vi "MoveMirror.vi"(1 "error in 2":errorcluster, 3 "POS X rad":dbl, 4 "POS Y rad":dbl) -> (0 "error out 2":errorcluster)   [LabVIEW 2011]
uses:
  Utilities/controls/ctlSeqFNs_PI_SysNr.ctl
  Variables/GlobalSetConfigurationPhysikalInstruments.vi
  Variables/GlobalSetNumberOfDigits_PhysikalInstruments.vi
  Variables/GlobalSetGetPositionParameters.vi
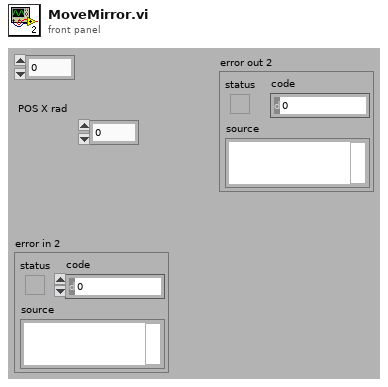
[diagram p1: front panel]
types:
  T1 = typedef "ctlSeqFNs_PI_SysNr.ctl" = enum16{"Zero", "E517", "E710"}
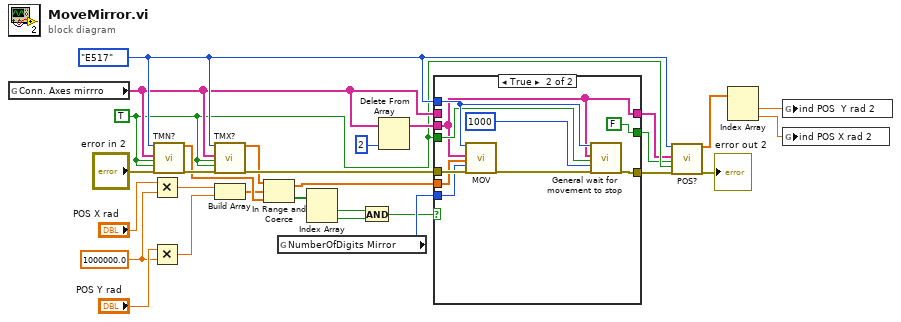
[diagram p0: block diagram]
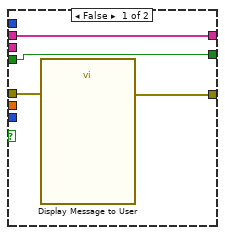
[diagram p2: hidden frame]
diagram:
  w15 = 1000000.0 ("y")
  w3 = TRUE ("All axes?")
  w9 = ctlSeqFNs_PI_SysNr."E517" ("DeviceNr.")
  n1 = global read "GlobalSetConfigurationPhysikalInstruments.vi" "Conn. Axes mirrro"() -> (w5:string[])
  n2 = Multiply(x="POS X rad", y=w15) -> (x*y=w13:dbl)
  n3 = Multiply(x="POS Y rad", y=w15) -> (x*y=w16:dbl)
  n4 = call "TMN?.vi"("System no."=w9, "Axes to query"=w5, "All axes?"=w3, "Axis identifier?"=w3, "error in"="error in 2") -> ("Minimum travel limit"=w25:dbl[], "error out"=w28:errorcluster)  [unwired: 13 in]
  n5 = call "TMX?.vi"("System no."=w9, "Axes to query"=w5, "All axes?"=w3, "Axis identifier?"=w3, "error in"=w28) -> ("Maximum travel limit"=w24:dbl[], "error out"=w27:errorcluster)  [unwired: 13 in]
  n6 = Build Array(w13, w16) -> (w23:dbl[])
  n7 = In Range and Coerce(upper limit=w24, x=w23, lower limit=w25) -> (coerced(x)=w18:dbl[], In Range?=w22:bool[])
  n8 = global read "GlobalSetNumberOfDigits_PhysikalInstruments.vi" "NumberOfDigits Mirror"() -> (w26:i32)
  n9 = Index Array(array=w22) -> (element #1=w21:bool, element #2=w20:bool)  [unwired: 2 in]
  n10 = And(x=w21, y=w20) -> (x .and. y?=w19:bool)
  n11 = Delete From Array(array=w5, index=2) -> (array with subset deleted=w6:string[])  [unwired: 1 in, 1 out]
  n12 = case shown="True" w19 {
    tunnel: w18 -> [_ w37]
    tunnel: w27 -> [w32 w43]
    tunnel: [w33 w41] -> w8
    tunnel: w6 -> [_ w35]
    tunnel: w9 -> [_ w40]
    tunnel: w26 -> [_ w38]
    tunnel: w5 -> [w31 _]
    tunnel: w3 -> [w30 w36]
    tunnel: [w31 w35] -> w2
    tunnel: [w30 FALSE] -> w1
    frame False {
      n13 = call "Display Message to User"("error in (no error)"=w32) -> ("error out"=w33:errorcluster)  [unwired: 9 in, 1 out]
    }
    frame True {
      n14 = call "MOV.vi"("System no."=w40, "Axes to move"=w35, "Position values"=w37, "No.of digits"=w38, "error in"=w43) -> ("error out"=w42:errorcluster)  [unwired: 14 in]
      n15 = call "General wait for movement to stop.vi"("System no."=w40, "Axes to wait for"=w35, "All axes?"=w36, "Additional wait time, ms"=u32 1000, "error in"=w42) -> ("error out"=w41:errorcluster)  [unwired: 13 in, 1 out]
    }
  }
  n16 = call "POS?.vi"("System no."=w9, "Axes to query"=w2, "All axes?"=w1, "Axis identifier?"=w3, "error in"=w8) -> ("Position"=w12:dbl[], "error out"=→"error out 2":errorcluster)  [unwired: 13 in]
  n17 = Index Array(array=w12) -> (element #1=w11:dbl, element #2=w10:dbl)  [unwired: 2 in]
  n18 = global write "GlobalSetGetPositionParameters.vi" "ind POS  Y rad 2"(w11) -> ()
  n19 = global write "GlobalSetGetPositionParameters.vi" "ind POS X rad 2"(w10) -> ()
